vi "Half Subtractor.vi"(2 "B":bool, 3 "A":bool) -> (0 "BORROW":bool, 1 "DIFF":bool)   [LabVIEW 2011]
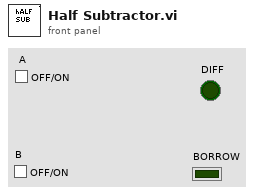
[diagram p1: front panel]
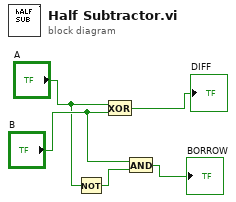
[diagram p0: block diagram]
diagram:
  n1 = Not(x="A") -> (.not. x?=w5:bool)
  n2 = Exclusive Or(1:"B", 2:"A") -> (0:→"DIFF":bool)
  n3 = And(x="B", y=w5) -> (x .and. y?=→"BORROW":bool)
